vi "x_pos_y_pos_int.vi"(0 "Image Out":T2(plugin-control), 1 "Calibrated Image":T2, 5 "ROI Descriptor":T7 {"Contours"."Type" items=["No Selection", "Point", "Line", "Rectangle", "Oval", "Polygon", "Free", "Annulus", "Unused2", "Unused3", "Broken Line", "Free Hand Line", "Rotated Rectangle"]}, 7 "Edge Options ROI 1":T5={"Edge Polarity"=2, "Kernel Size"=5, "Width"=5, "Minimum Edge Strength"=50.0, "Interpolation Type"=enum."Bilinear Fixed", "Data Processing Method"=enum."Average"} {"Edge Polarity" items=["All Edges", "Rising Edges", "Falling Edges"]; "Minimum Edge Strength" format="%.2f"; "Width" step=2; "Kernel Size" step=2}, 9 "Search Direction ROI 1":u32(ring) items=["Left to Right", "Right to Left", "Top to Bottom", "Bottom to Top"], 11 "error in (no error)":errorcluster, 12 "Line Options ROI 1":T3={"Number of Lines"=1, "Type"=enum."Best Edge Rake", "Min. Score"=10.0, "Max. Score"=1000.0, "Orientation"=0.0, "Angle Range"=10.0, "Angle Tolerance"=1.0, "Step Size"=10, "Min. SNR (db)"=0.0, "Min. Points (%)"=25.0, "Hough Iterations"=5} {"Min. Points (%)" min=0.0 max=100.0; "Min. SNR (db)" min=0.0; "Max. Score" min=0.0 max=1024.0; "Min. Score" min=0.0 max=1024.0 step=1.0}, 13 "OverlayOptions":T1) -> (4 "Position":sgl, 15 "error out":errorcluster)   [LabVIEW 2019, in "Algorithm.lvclass"]
uses:
  FrameworkOverrides/Algorithm.lvclass
  <vilib>/vision/NI_Vision_Development_Module.lvlib
  <vilib>/vision/Measure.llb/Edge Polarity.ctl
  <vilib>/vision/Measure.llb/Edge Options.ctl
  <vilib>/vision/Measure.llb/Straight Edge Process.ctl
  <vilib>/vision/Measure.llb/Straight Edge Options.ctl
  <vilib>/vision/Image Controls.llb/IMAQ Image.ctl
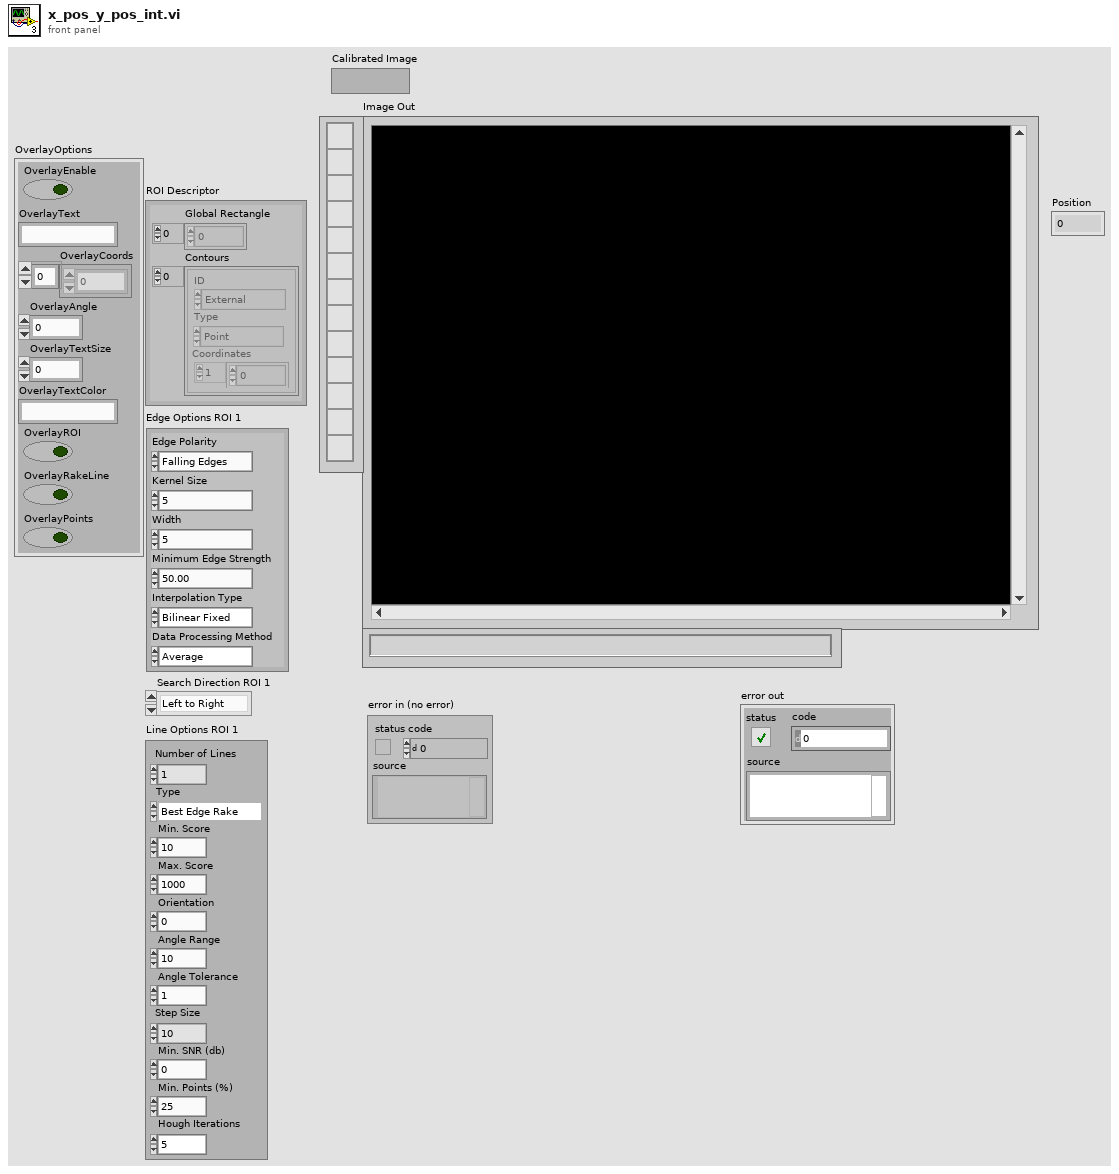
[diagram p1: front panel]
types:
  T1 = cluster{"OverlayEnable":bool, "OverlayText":string, "OverlayCoords":i32[], "OverlayAngle":i32, "OverlayTextSize":i32, "OverlayTextColor":string, "OverlayROI":bool, "OverlayRakeLine":bool, "OverlayPoints":bool}
  T2 = typedef "IMAQ Image.ctl" = refnum<image>
  T3 = typedef "Straight Edge Options.ctl" = cluster{"Number of Lines":i32, "Type":T4, "Min. Score":dbl, "Max. Score":dbl, "Orientation":dbl, "Angle Range":dbl, "Angle Tolerance":dbl, "Step Size":u32, "Min. SNR (db)":dbl, "Min. Points (%)":dbl, "Hough Iterations":i32}
  T4 = typedef "Straight Edge Process.ctl" = enum32{"First Edge Rake", "Best Edge Rake", "Hough Edge Rake", "First Edge Projection", "Best Edge Projection"}
  T5 = typedef "Edge Options.ctl" = cluster{"Edge Polarity":T6, "Kernel Size":u32, "Width":u32, "Minimum Edge Strength":sgl, "Interpolation Type":enum32{"Zero Order", "Bilinear", "Quadratic", "Cubic", "Bilinear Fixed"}, "Data Processing Method":enum32{"Average", "Median"}}
  T6 = typedef "Edge Polarity.ctl" = u32
  T7 = cluster{"Global Rectangle":i32[], "Contours":cluster{"ID":enum32{"External", "Internal"}, "Type":u32, "Coordinates":i32[]}[]}
  T8 = cluster{"Point1 (Pixels)":cluster{"X":sgl, "Y":sgl}, "Point2 (Pixels)":cluster{"X":sgl, "Y":sgl}, "Point1 (Real-World)":cluster{"X":sgl, "Y":sgl}, "Point2 (Real-World)":cluster{"X":sgl, "Y":sgl}, "Angle (Pixel)":dbl, "Angle (Real-World)":dbl, "Score":dbl, "Straightness":dbl, "Average SNR (db)":dbl, "Calibration Valid":bool}[]
  T9 = typedef "Search Line.ctl" = cluster{"Start Point":cluster{"X":sgl, "Y":sgl}, "End Point":cluster{"X":sgl, "Y":sgl}, "Edge Info":T10[], "Edge Map":dbl[], "Calibration Valid":bool}
  T10 = typedef "Edge New.ctl" = cluster{"Location (Pixel)":cluster{"X":sgl, "Y":sgl}, "Location (Real-World)":cluster{"X":sgl, "Y":sgl}, "Distance (Pixel)":dbl, "Distance (Real-World)":dbl, "Strength":dbl, "Noise":dbl, "Rising?":bool}
  T11 = cluster{"Point1 (Pixels)":cluster{"X":sgl, "Y":sgl}, "Point2 (Pixels)":cluster{"X":sgl, "Y":sgl}, "Point1 (Real-World)":cluster{"X":sgl, "Y":sgl}, "Point2 (Real-World)":cluster{"X":sgl, "Y":sgl}, "Angle (Pixel)":dbl, "Angle (Real-World)":dbl, "Score":dbl, "Straightness":dbl, "Average SNR (db)":dbl, "Calibration Valid":bool}
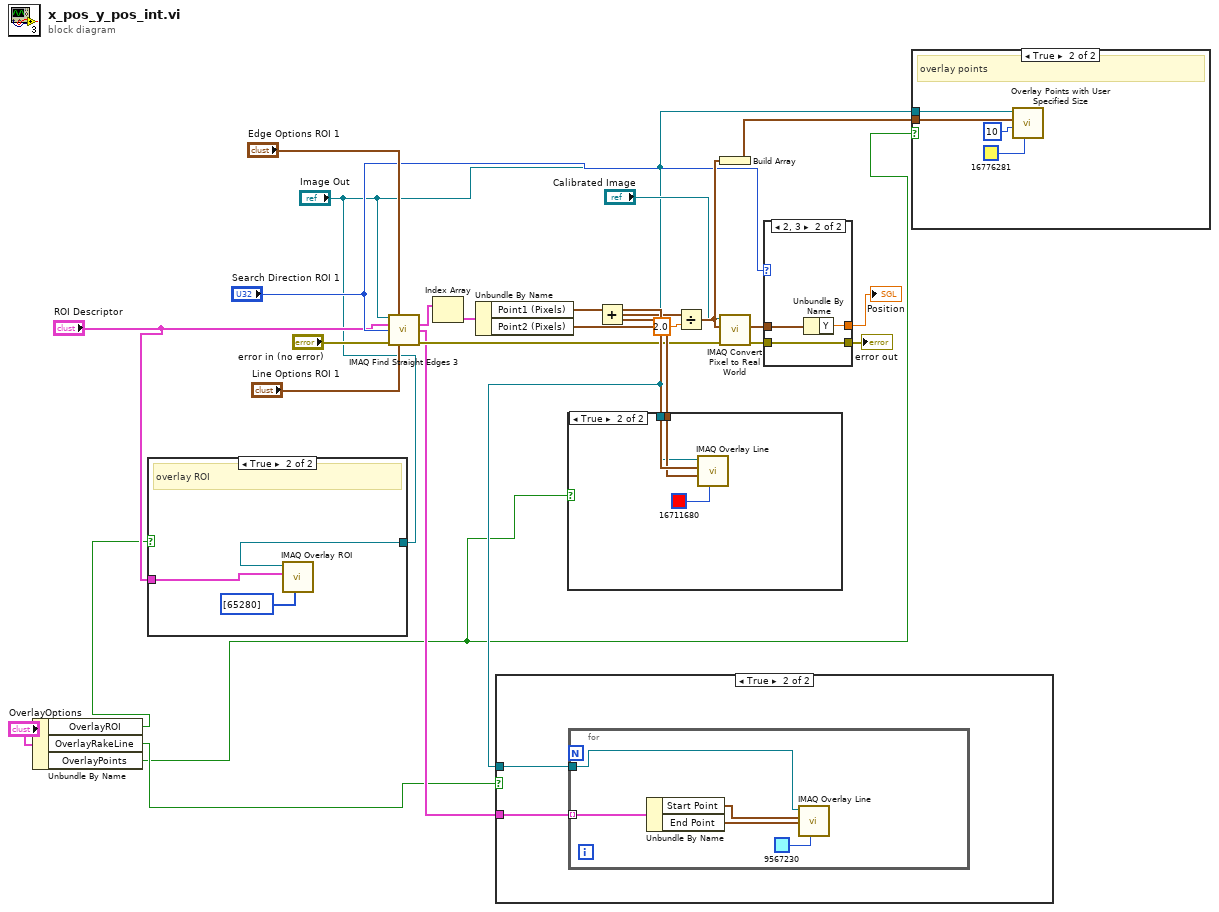
[diagram p0: block diagram]
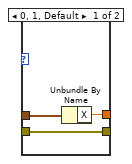
[diagram p6: hidden frame]
diagram:
  n1 = Unbundle By Name("OverlayOptions") -> ("OverlayROI"=w3:bool, "OverlayRakeLine"=w2:bool, "OverlayPoints"=w1:bool)
  n2 = case shown="True" w3 {
    tunnel: "ROI Descriptor" -> [_ w28]
    tunnel: "Image Out" -> [_ w27]
    frame False {
    }
    frame True {
      # "overlay ROI"
      n3 = call "IMAQ Overlay ROI"("Colors (Green)"=u32[] [65280], "ROI Descriptor"=w28, "Image"=w27) -> ()  [unwired: 7 in, 2 out]
    }
  }
  n4 = call "IMAQ Find Straight Edges 3"("Image"="Image Out", "Edge Options"="Edge Options ROI 1", "ROI Descriptor"="ROI Descriptor", "Search Direction"="Search Direction ROI 1", "error in (no error)"="error in (no error)", "Line Options"="Line Options ROI 1") -> ("Straight Edges"=w23:T8, "Search Lines Information"=w6:T9[], "error out"=w12:errorcluster)  [unwired: 5 in, 2 out]
  n5 = Index Array(array=w23) -> (element=w22:T11)  [unwired: 1 in]
  n6 = Unbundle By Name(w22) -> ("Point1 (Pixels)"=w21:cluster{"X":sgl, "Y":sgl}, "Point2 (Pixels)"=w20:cluster{"X":sgl, "Y":sgl})
  n7 = case shown="True" w2 {
    tunnel: w6 -> [_ w30]
    tunnel: "Image Out" -> [_ w29]
    frame False {
    }
    frame True {
      n8 = for {
        tunnel: w30 -> [w35] mode=indexing
        tunnel: w29 -> [w32]
        n9 = Unbundle By Name(w35) -> ("Start Point"=w34:cluster{"X":sgl, "Y":sgl}, "End Point"=w33:cluster{"X":sgl, "Y":sgl})
        n10 = call "IMAQ Overlay Line"("Color"=u32 9567230, "End Point"=w33, "Start Point"=w34, "Image"=w32) -> ()  [unwired: 6 in, 2 out]
      }
    }
  }
  n11 = case shown="True" w1 {
    tunnel: w21 -> [_ w38]
    tunnel: w20 -> [_ w37]
    tunnel: "Image Out" -> [_ w36]
    frame False {
      # "Overlay Line"
    }
    frame True {
      n12 = call "IMAQ Overlay Line"("Color"=u32 16711680, "End Point"=w37, "Start Point"=w38, "Image"=w36) -> ()  [unwired: 6 in, 2 out]
    }
  }
  n13 = Add(x=w21, y=w20) -> (x+y=w19:cluster{"X":sgl, "Y":sgl})
  n14 = Divide(x=w19, y=2.0) -> (x/y=w16:cluster{"X":dbl, "Y":dbl})
  n15 = Build Array(w16) -> (w17:cluster{"X":dbl, "Y":dbl}[])
  n16 = call "IMAQ Convert Pixel to Real World"("error in (no error)"=w12, "Pixel Coordinates"=w16, "Calibrated Image"="Calibrated Image") -> ("error out"=w11:errorcluster, "Real World Coordinates"=w14:cluster{"X":sgl, "Y":sgl})  [unwired: 3 in, 4 out]
  n17 = case shown="2, 3" "Search Direction ROI 1" {
    tunnel: w14 -> [w42 w45]
    tunnel: [w41 w44] -> w13
    tunnel: w11 -> [w40 w43]
    tunnel: [w40 w43] -> w8
    frame 0, 1, Default {
      n18 = Unbundle By Name(w42) -> ("X"=w41:sgl)
    }
    frame 2, 3 {
      n19 = Unbundle By Name(w45) -> ("Y"=w44:sgl)
    }
  }
  "Position" <- w13
  "error out" <- w8
  n20 = case shown="True" w1 {
    tunnel: w17 -> [_ w49]
    tunnel: "Image Out" -> [_ w48]
    frame False {
    }
    frame True {
      # "overlay points"
      n21 = call "Overlay Points with User Specified Size.vi"("Color"=u32 16776281, "Point Diameter (5)"=u32 10, "Points"=w49, "Image In"=w48) -> ()  [unwired: 6 in, 2 out]
    }
  }
